vi "TMP007.vi"(8 "i_error":errorcluster, 10 "i_Ref":T1={"Adress"=19, "CMD"=enum."#0 V_Sensor", "i_Value"=0, "R/W"=enum."Read"} {"i_Value" format="%.0b"; "Adress" format="%02x"}) -> (0 "o_error":errorcluster, 2 "Bytes Read":u8[](array[numeric]))   [LabVIEW 2016]
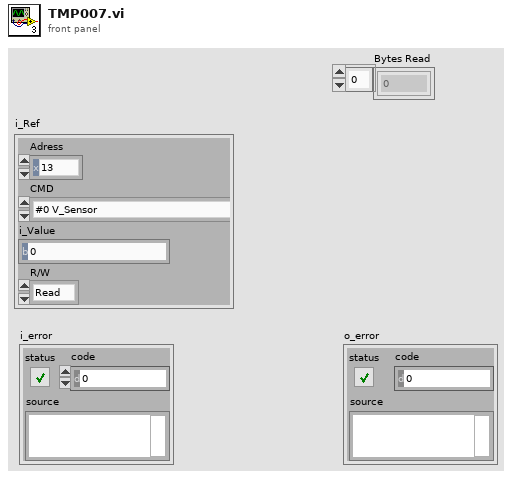
[diagram p1: front panel]
types:
  T1 = cluster{"Adress":u8, "CMD":enum8{"#0 V_Sensor", "#1 T_Die", "#2 Configuration", "#3 T_Obj", "#4 Status", "#5 Status mask and enable", "#6 T_Obj high limit", "#7 T_Obj low-limit", "#8 T_Die high-limit", "#9 T_Die low-limit", "#0A S0 coefficient ", "#0B A1 Coefficient", "#0C A2 Coefficient", "#0D B0 Coefficient", "#0E B1 Coefficient", "#0F B2Coefficient", "#10 C2 Coefficient", "#11 TC0 Coefficientd", "#12 TC1 Coefficient", "#1E Manufacturer ID", "#1F Device ID", "#2A Memory access"}, "i_Value":u16, "R/W":enum16{"Read", "Write"}}
  T2 = enum8{"#0 V_Sensor", "#1 T_Die", "#2 Configuration", "#3 T_Obj", "#4 Status", "#5 Status mask and enable", "#6 T_Obj high limit", "#7 T_Obj low-limit", "#8 T_Die high-limit", "#9 T_Die low-limit", "#0A S0 coefficient ", "#0B A1 Coefficient", "#0C A2 Coefficient", "#0D B0 Coefficient", "#0E B1 Coefficient", "#0F B2Coefficient", "#10 C2 Coefficient", "#11 TC0 Coefficientd", "#12 TC1 Coefficient", "#1E Manufacturer ID", "#1F Device ID", "#2A Memory access"}
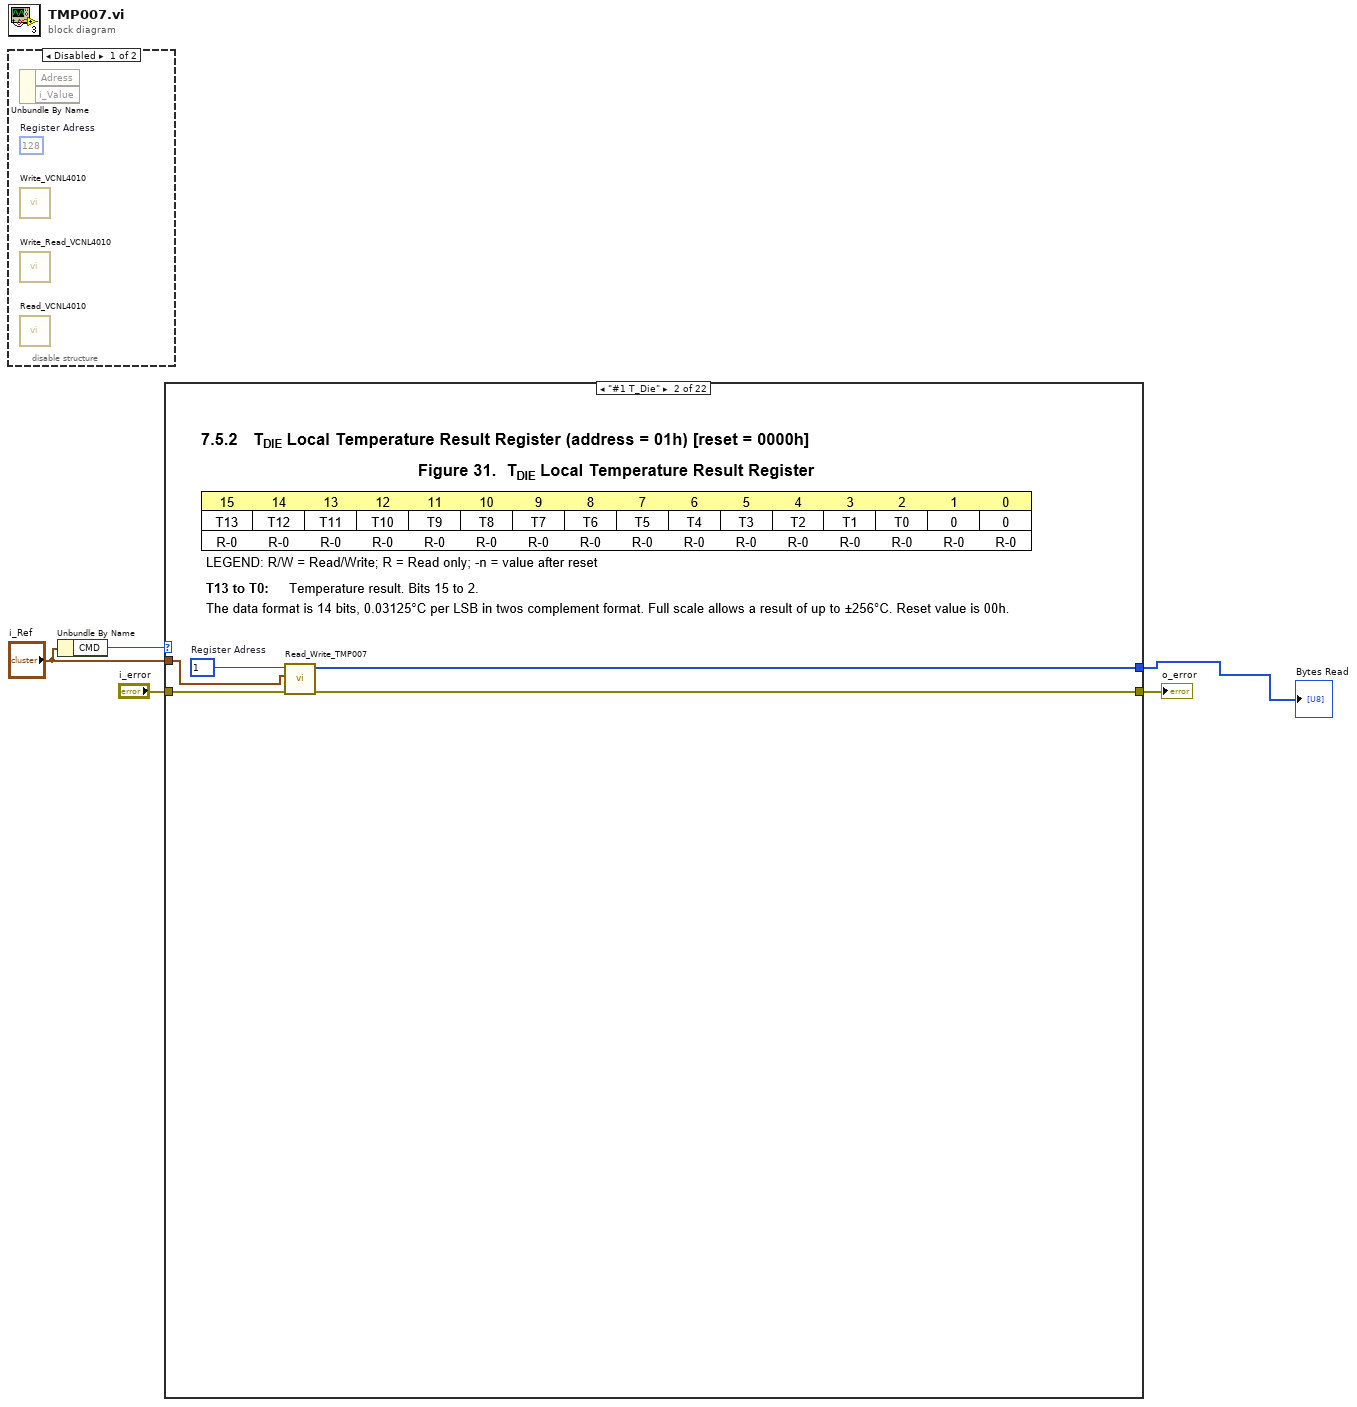
[diagram p0: block diagram]
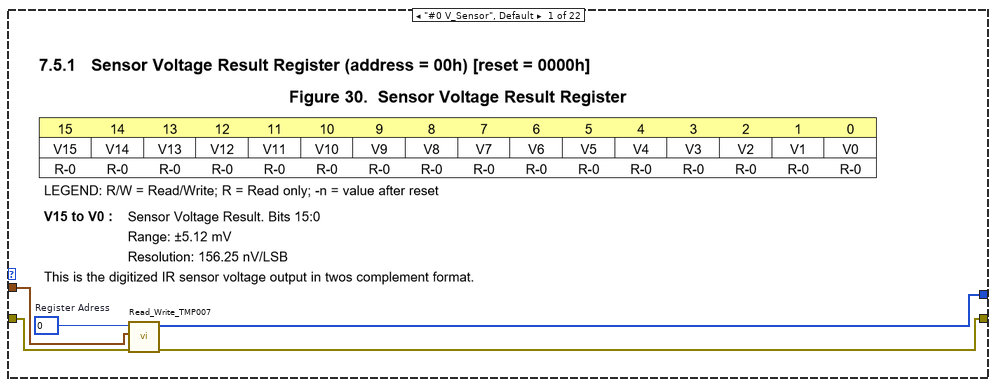
[diagram p2: hidden frame]
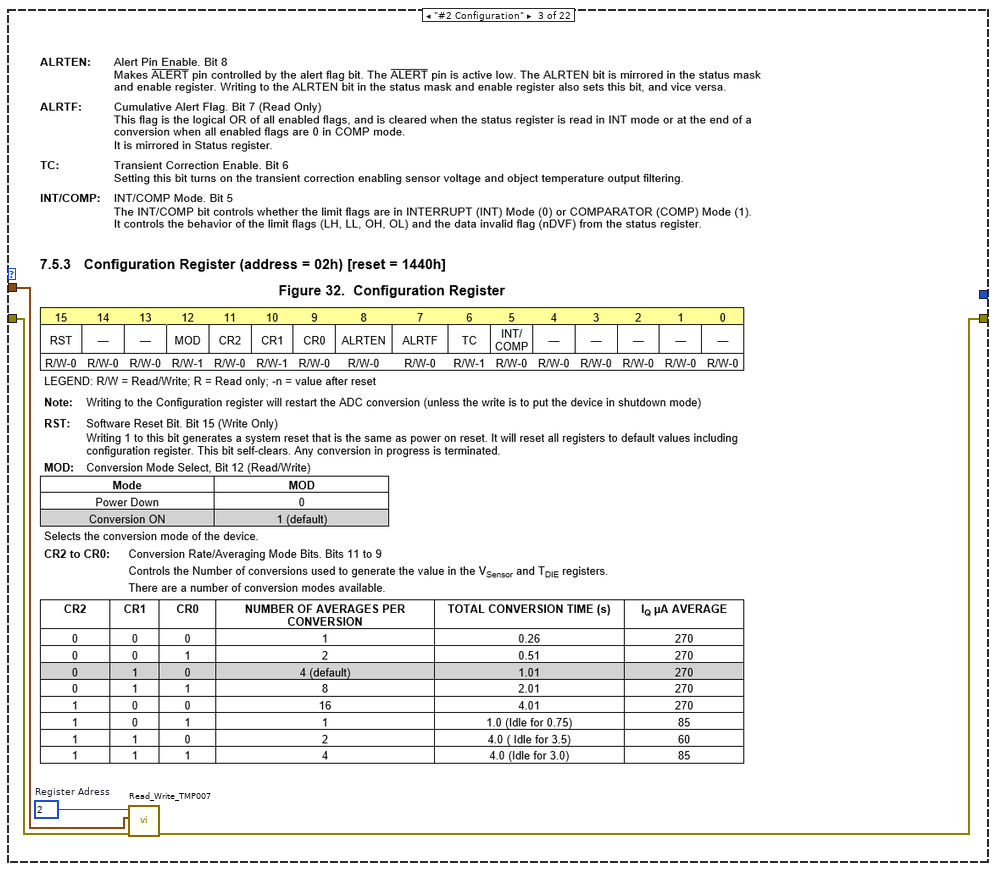
[diagram p3: hidden frame]
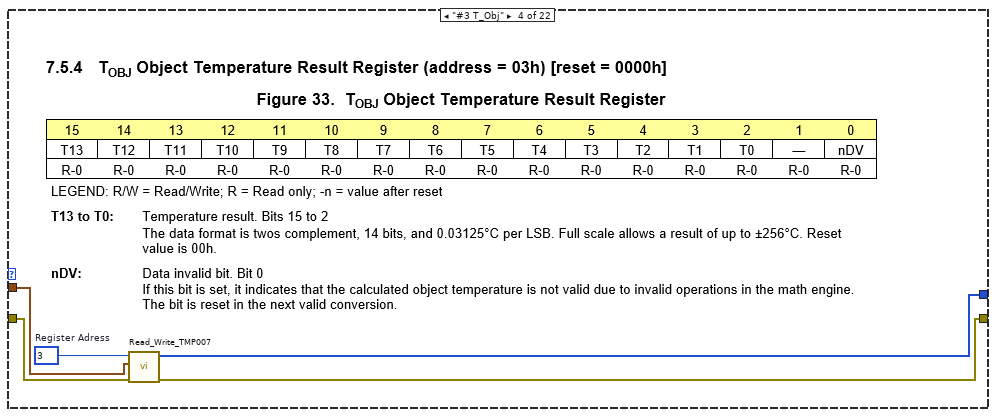
[diagram p4: hidden frame]
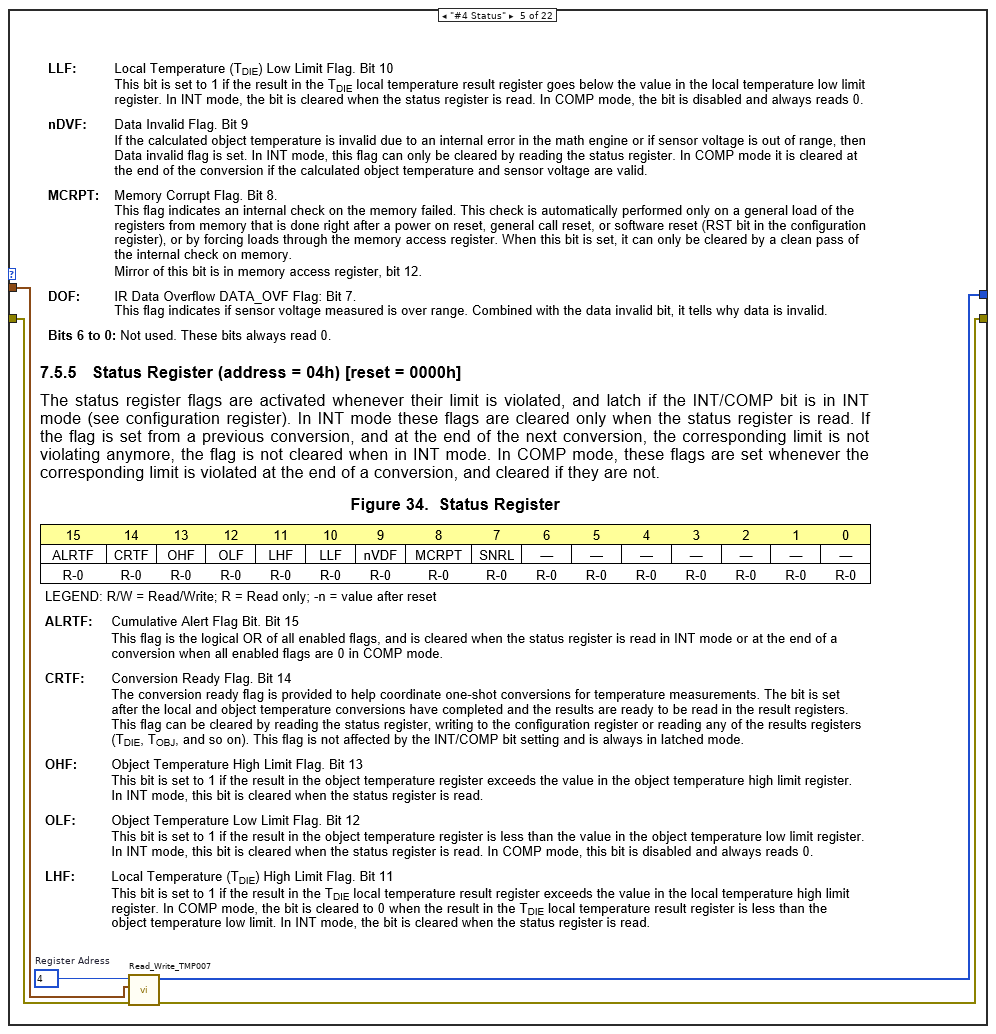
[diagram p5: hidden frame]
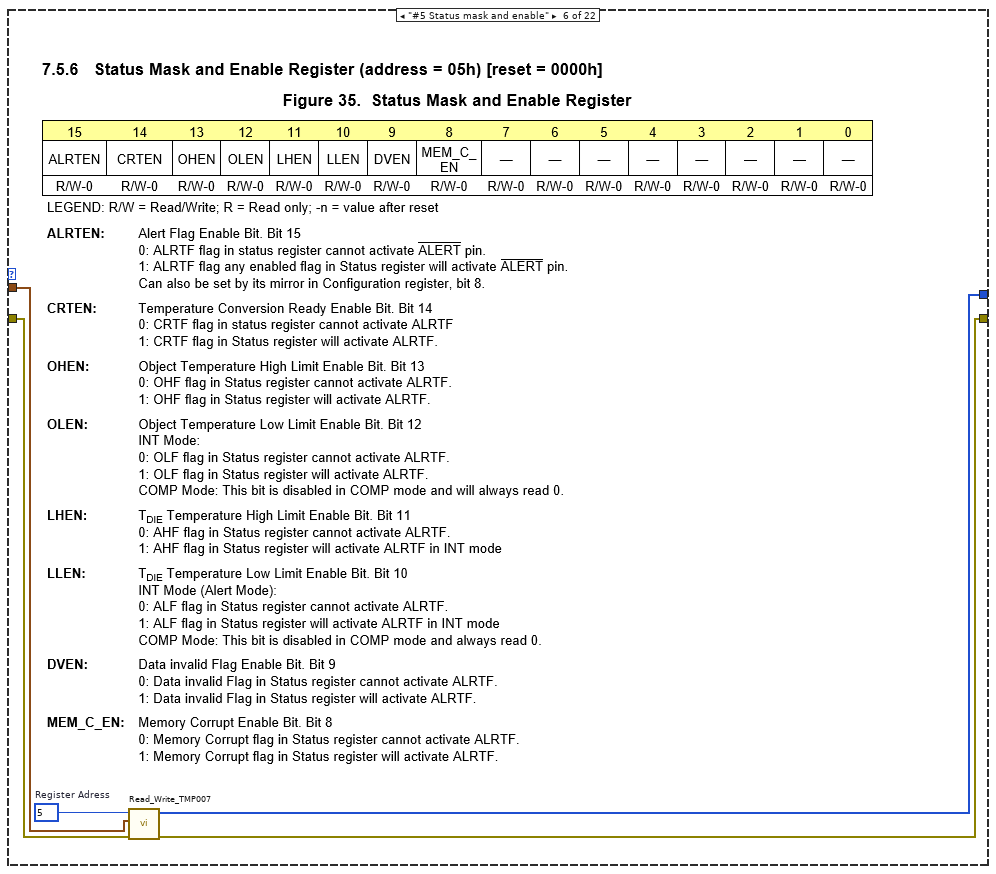
[diagram p6: hidden frame]
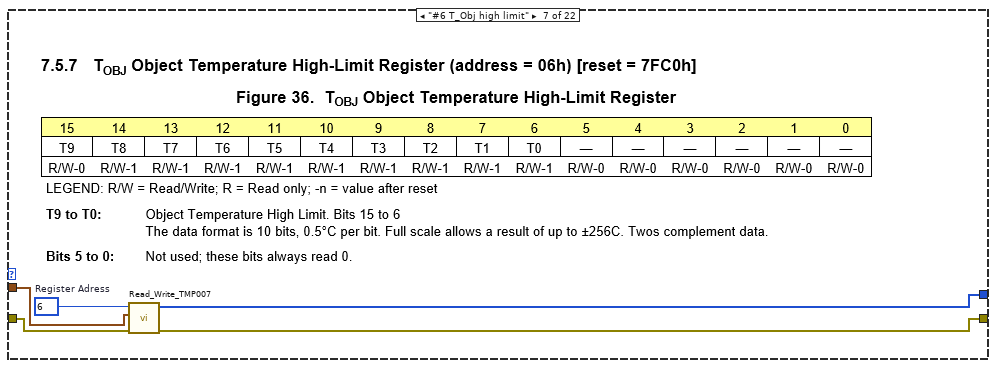
[diagram p7: hidden frame]
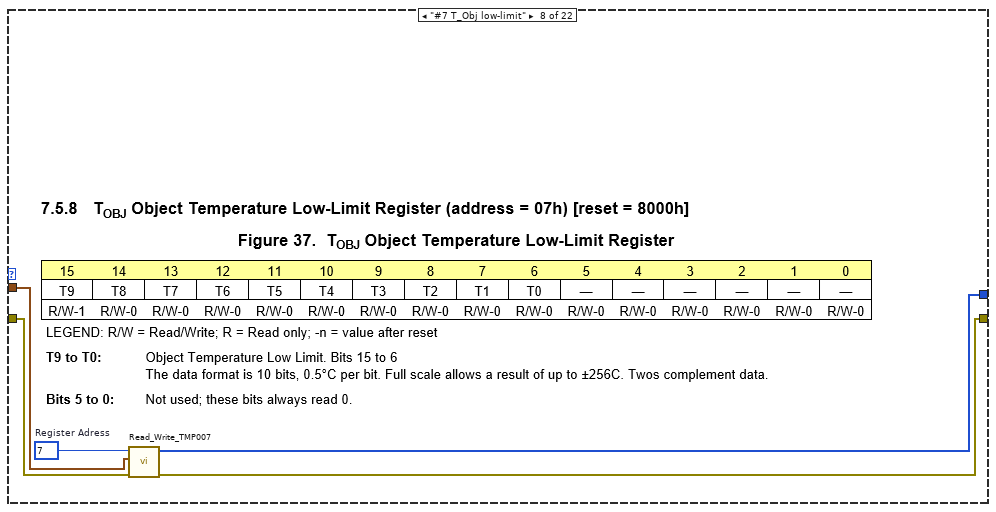
[diagram p8: hidden frame]
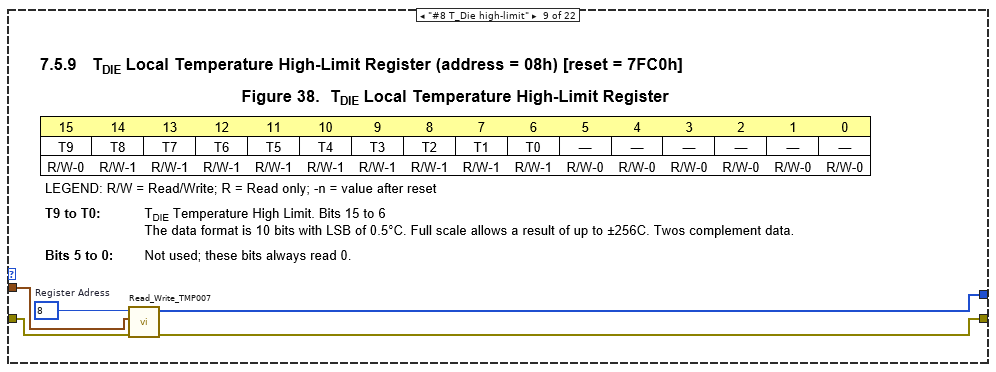
[diagram p9: hidden frame]
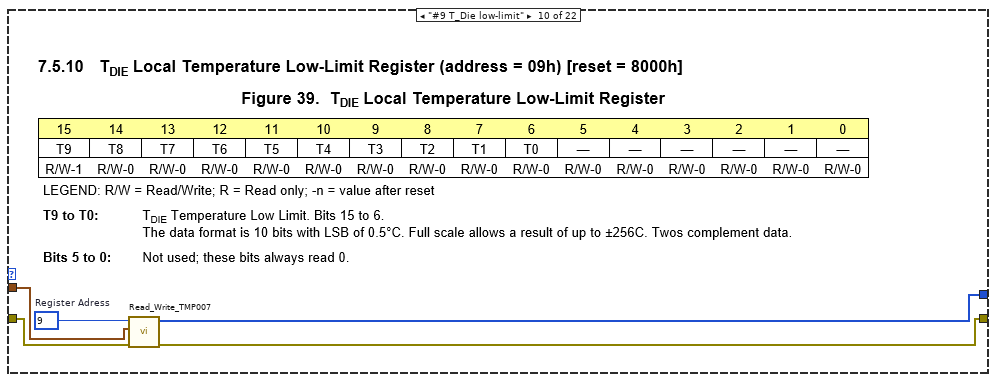
[diagram p10: hidden frame]
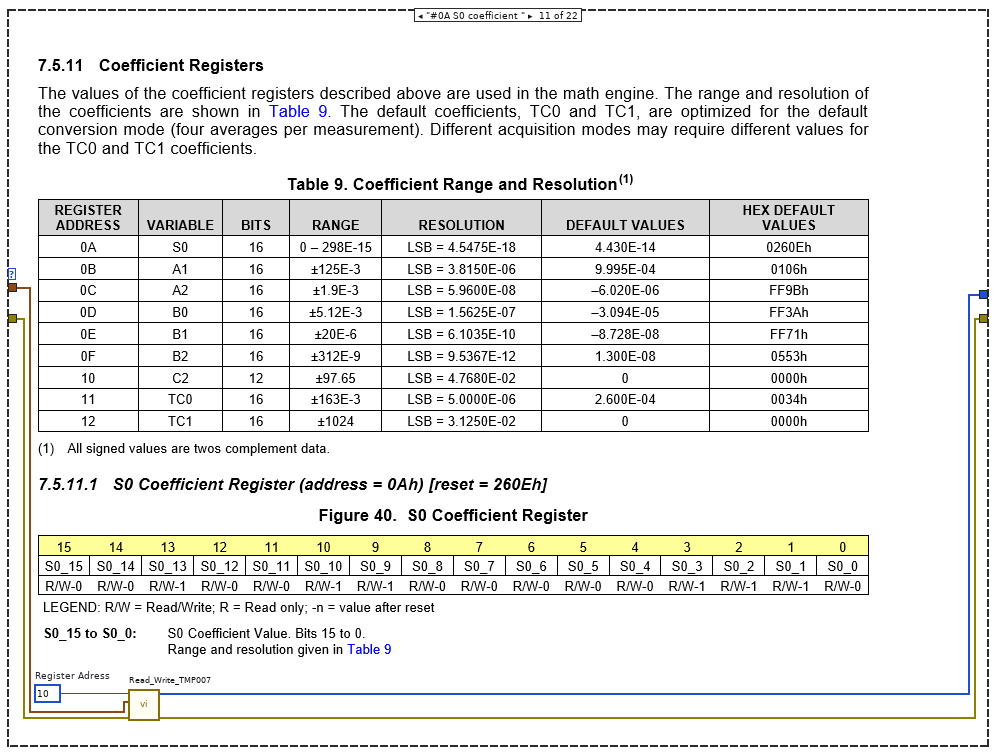
[diagram p11: hidden frame]
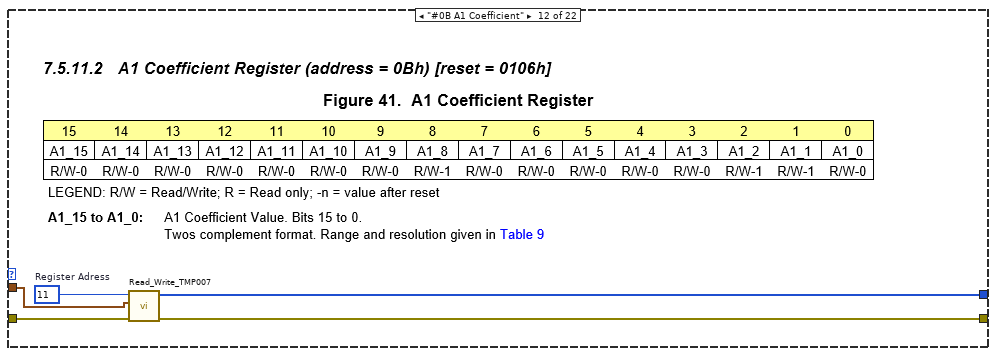
[diagram p12: hidden frame]
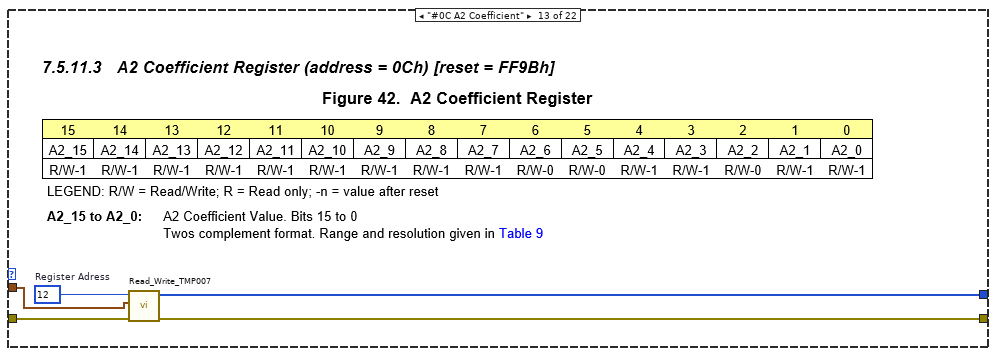
[diagram p13: hidden frame]
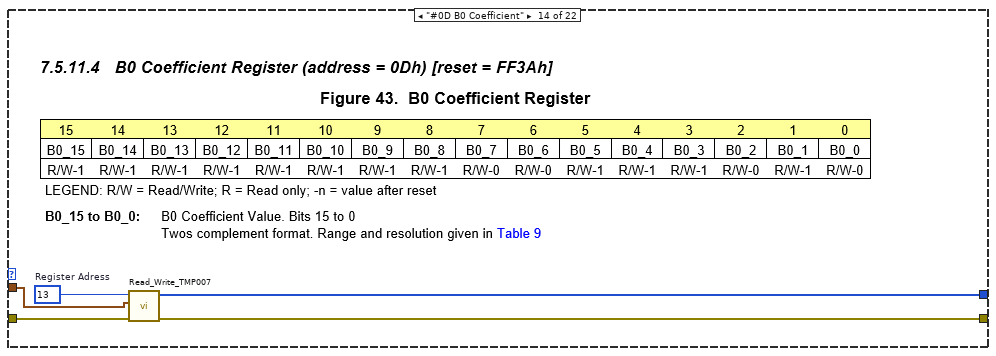
[diagram p14: hidden frame]
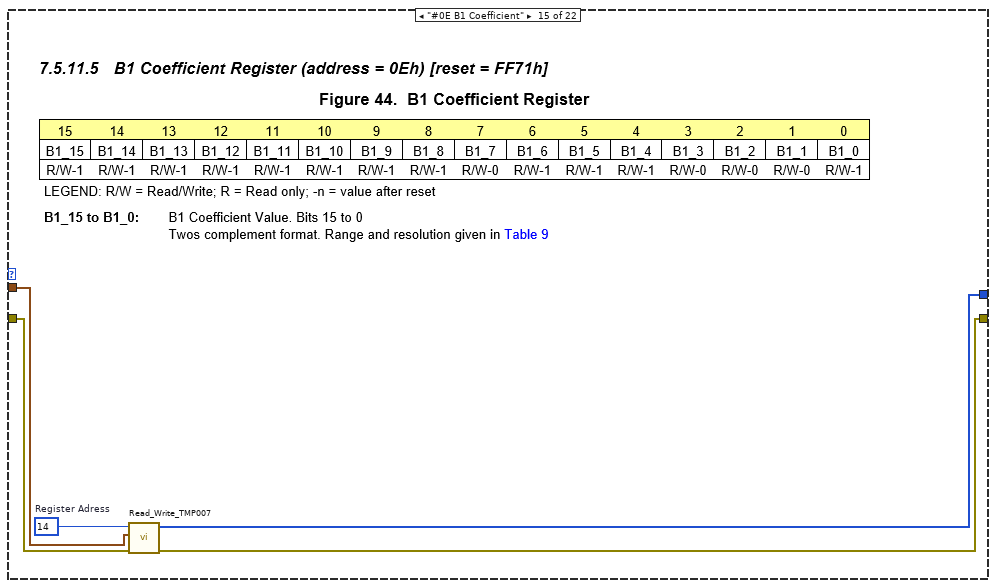
[diagram p15: hidden frame]
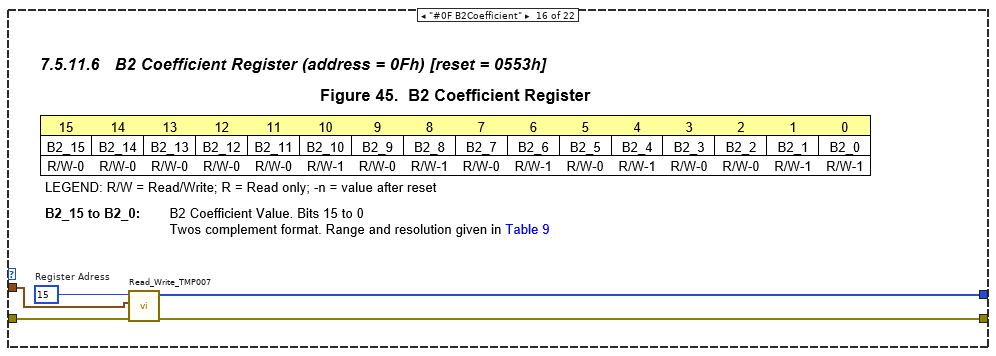
[diagram p16: hidden frame]
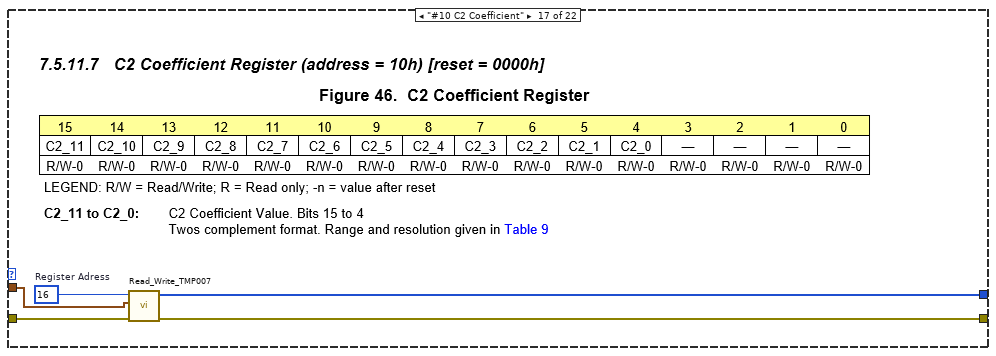
[diagram p17: hidden frame]
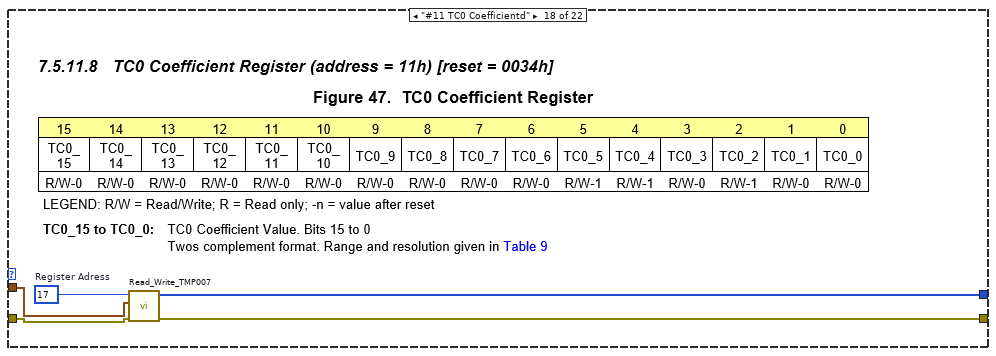
[diagram p18: hidden frame]
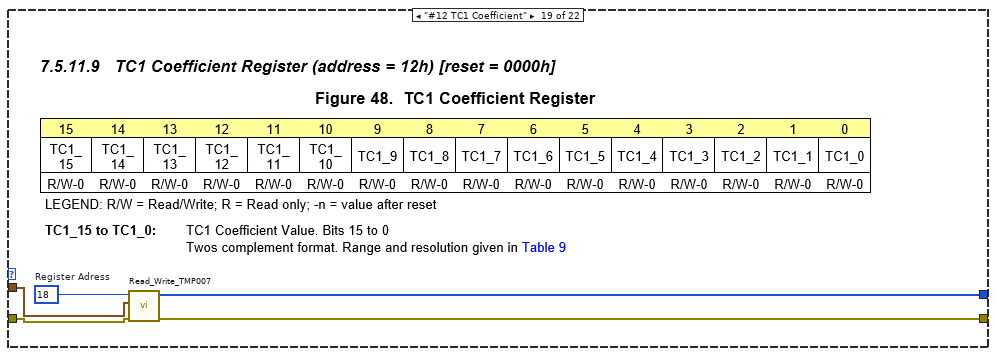
[diagram p19: hidden frame]
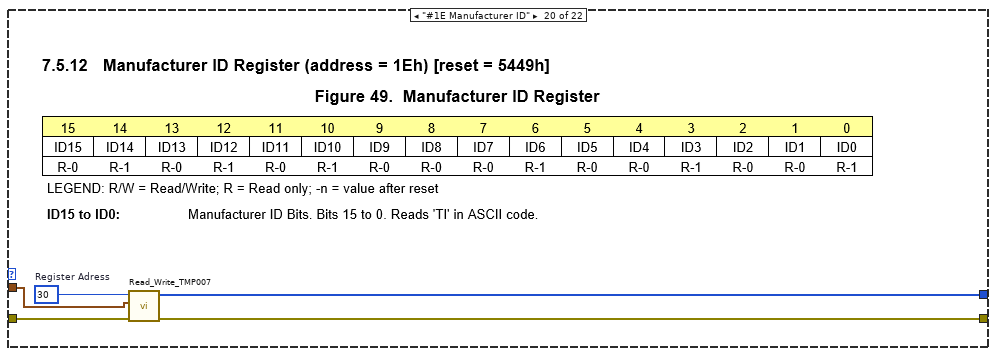
[diagram p20: hidden frame]
diagram:
  n1 = disable-structure shown="Disabled" {
    frame Disabled {
      (unwired) 128  # Register Adress
      n2 = Unbundle By Name() -> ()  [unwired: 1 in, 2 out]
      n3 = call "Write_VCNL4010.vi"() -> ()  [unwired: 11 in, 1 out]
      n4 = call "Write_Read_VCNL4010.vi"() -> ()  [unwired: 10 in, 2 out]
      n5 = call "Read_VCNL4010.vi"() -> ()  [unwired: 10 in, 2 out]
    }
    frame Enabled {
    }
  }
  n6 = Unbundle By Name("i_Ref") -> ("CMD"=w2:T2)
  n7 = case shown="\"#1 T_Die\"" w2 {
    tunnel: "i_Ref" -> [w9 w14 w17 w22 w27 w33 w37 w43 w48 w52 w58 w63 w68 w73 w79 w81 w88 w92 w97 w103 w108 w111]
    tunnel: [w6 w11 _ w21 w26 w30 w36 w40 w45 w51 w55 w61 w65 w70 w75 w82 w85 w90 w95 w101 w105 w112] -> w1
    tunnel: "i_error" -> [w8 w13 w18 w24 w29 w32 w38 w42 w47 w53 w57 w62 w67 w72 w77 w84 w87 w93 w98 w104 w107 w114]
    tunnel: [w7 w12 w16 w20 w25 w31 w35 w41 w46 w50 w56 w60 w66 w71 w76 w83 w86 w94 w99 w102 w106 w113] -> w3
    frame "#0 V_Sensor", Default {
      w10 = u8 0  # Register Adress
      n8 = call "Read_Write_TMP007.vi"("error in (no error)"=w8, "i_Ref"=w9, "Register Adress"=w10) -> ("error out"=w7:errorcluster, "Bytes Read"=w6:u8[])  [unwired: 7 in]
    }
    frame "#1 T_Die" {
      w15 = u8 1  # Register Adress
      n9 = call "Read_Write_TMP007.vi"("error in (no error)"=w13, "i_Ref"=w14, "Register Adress"=w15) -> ("error out"=w12:errorcluster, "Bytes Read"=w11:u8[])  [unwired: 7 in]
    }
    frame "#2 Configuration" {
      w19 = u8 2  # Register Adress
      n10 = call "Read_Write_TMP007.vi"("error in (no error)"=w18, "i_Ref"=w17, "Register Adress"=w19) -> ("error out"=w16:errorcluster)  [unwired: 7 in, 1 out]
    }
    frame "#3 T_Obj" {
      w23 = u8 3  # Register Adress
      n11 = call "Read_Write_TMP007.vi"("error in (no error)"=w24, "i_Ref"=w22, "Register Adress"=w23) -> ("error out"=w20:errorcluster, "Bytes Read"=w21:u8[])  [unwired: 7 in]
    }
    frame "#4 Status" {
      w28 = u8 4  # Register Adress
      n12 = call "Read_Write_TMP007.vi"("error in (no error)"=w29, "i_Ref"=w27, "Register Adress"=w28) -> ("error out"=w25:errorcluster, "Bytes Read"=w26:u8[])  [unwired: 7 in]
    }
    frame "#5 Status mask and enable" {
      w34 = u8 5  # Register Adress
      n13 = call "Read_Write_TMP007.vi"("error in (no error)"=w32, "i_Ref"=w33, "Register Adress"=w34) -> ("error out"=w31:errorcluster, "Bytes Read"=w30:u8[])  [unwired: 7 in]
    }
    frame "#6 T_Obj high limit" {
      w39 = u8 6  # Register Adress
      n14 = call "Read_Write_TMP007.vi"("error in (no error)"=w38, "i_Ref"=w37, "Register Adress"=w39) -> ("error out"=w35:errorcluster, "Bytes Read"=w36:u8[])  [unwired: 7 in]
    }
    frame "#7 T_Obj low-limit" {
      w44 = u8 7  # Register Adress
      n15 = call "Read_Write_TMP007.vi"("error in (no error)"=w42, "i_Ref"=w43, "Register Adress"=w44) -> ("error out"=w41:errorcluster, "Bytes Read"=w40:u8[])  [unwired: 7 in]
    }
    frame "#8 T_Die high-limit" {
      w49 = u8 8  # Register Adress
      n16 = call "Read_Write_TMP007.vi"("error in (no error)"=w47, "i_Ref"=w48, "Register Adress"=w49) -> ("error out"=w46:errorcluster, "Bytes Read"=w45:u8[])  [unwired: 7 in]
    }
    frame "#9 T_Die low-limit" {
      w54 = u8 9  # Register Adress
      n17 = call "Read_Write_TMP007.vi"("error in (no error)"=w53, "i_Ref"=w52, "Register Adress"=w54) -> ("error out"=w50:errorcluster, "Bytes Read"=w51:u8[])  [unwired: 7 in]
    }
    frame "#0A S0 coefficient " {
      w59 = u8 10  # Register Adress
      n18 = call "Read_Write_TMP007.vi"("error in (no error)"=w57, "i_Ref"=w58, "Register Adress"=w59) -> ("error out"=w56:errorcluster, "Bytes Read"=w55:u8[])  [unwired: 7 in]
    }
    frame "#0B A1 Coefficient" {
      w64 = u8 11  # Register Adress
      n19 = call "Read_Write_TMP007.vi"("error in (no error)"=w62, "i_Ref"=w63, "Register Adress"=w64) -> ("error out"=w60:errorcluster, "Bytes Read"=w61:u8[])  [unwired: 7 in]
    }
    frame "#0C A2 Coefficient" {
      w69 = u8 12  # Register Adress
      n20 = call "Read_Write_TMP007.vi"("error in (no error)"=w67, "i_Ref"=w68, "Register Adress"=w69) -> ("error out"=w66:errorcluster, "Bytes Read"=w65:u8[])  [unwired: 7 in]
    }
    frame "#0D B0 Coefficient" {
      w74 = u8 13  # Register Adress
      n21 = call "Read_Write_TMP007.vi"("error in (no error)"=w72, "i_Ref"=w73, "Register Adress"=w74) -> ("error out"=w71:errorcluster, "Bytes Read"=w70:u8[])  [unwired: 7 in]
    }
    frame "#0E B1 Coefficient" {
      w78 = u8 14  # Register Adress
      n22 = call "Read_Write_TMP007.vi"("error in (no error)"=w77, "i_Ref"=w79, "Register Adress"=w78) -> ("error out"=w76:errorcluster, "Bytes Read"=w75:u8[])  [unwired: 7 in]
    }
    frame "#0F B2Coefficient" {
      w80 = u8 15  # Register Adress
      n23 = call "Read_Write_TMP007.vi"("error in (no error)"=w84, "i_Ref"=w81, "Register Adress"=w80) -> ("error out"=w83:errorcluster, "Bytes Read"=w82:u8[])  [unwired: 7 in]
    }
    frame "#10 C2 Coefficient" {
      w89 = u8 16  # Register Adress
      n24 = call "Read_Write_TMP007.vi"("error in (no error)"=w87, "i_Ref"=w88, "Register Adress"=w89) -> ("error out"=w86:errorcluster, "Bytes Read"=w85:u8[])  [unwired: 7 in]
    }
    frame "#11 TC0 Coefficientd" {
      w91 = u8 17  # Register Adress
      n25 = call "Read_Write_TMP007.vi"("error in (no error)"=w93, "i_Ref"=w92, "Register Adress"=w91) -> ("error out"=w94:errorcluster, "Bytes Read"=w90:u8[])  [unwired: 7 in]
    }
    frame "#12 TC1 Coefficient" {
      w96 = u8 18  # Register Adress
      n26 = call "Read_Write_TMP007.vi"("error in (no error)"=w98, "i_Ref"=w97, "Register Adress"=w96) -> ("error out"=w99:errorcluster, "Bytes Read"=w95:u8[])  [unwired: 7 in]
    }
    frame "#1E Manufacturer ID" {
      w100 = u8 30  # Register Adress
      n27 = call "Read_Write_TMP007.vi"("error in (no error)"=w104, "i_Ref"=w103, "Register Adress"=w100) -> ("error out"=w102:errorcluster, "Bytes Read"=w101:u8[])  [unwired: 7 in]
    }
    frame "#1F Device ID" {
      w109 = u8 31  # Register Adress
      n28 = call "Read_Write_TMP007.vi"("error in (no error)"=w107, "i_Ref"=w108, "Register Adress"=w109) -> ("error out"=w106:errorcluster, "Bytes Read"=w105:u8[])  [unwired: 7 in]
    }
    frame "#2A Memory access" {
      w110 = u8 42  # Register Adress
      n29 = call "Read_Write_TMP007.vi"("error in (no error)"=w114, "i_Ref"=w111, "Register Adress"=w110) -> ("error out"=w113:errorcluster, "Bytes Read"=w112:u8[])  [unwired: 7 in]
    }
  }
  "o_error" <- w3
  "Bytes Read" <- w1
